vi "编码输出.vi"(8 "error in (no error)":errorcluster, 11 "SingleStepTestV3输入":refnum<class "SingleStepTestV2.lvclass">) -> (0 "error out":errorcluster, 3 "SingleStepTestV3输出":refnum<class "SingleStepTestV2.lvclass">)   [LabVIEW 2016, in "SingleStepTestV2.lvlib" / "SingleStepTestV2.lvclass"]
uses:
  SingleStepTestV2.lvclass
  SingleStepTestV2.lvclass/SingleStepTestV2.ctl
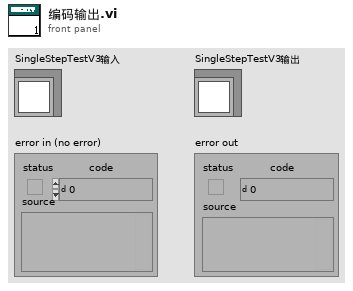
[diagram p1: front panel]
types:
  T1 = typedef "SingleStepTestV2.lvclass/State Data.ctl" = cluster{"data":u16[]}
  T2 = typedef "SingleStepTestV2.lvclass/控温操作.ctl" = enum32{"未选择", "控温开", "控温关"}
  T3 = typedef "SingleStepTestV3.lvclass/注射泵操作.ctl" = enum32{"复位", "注入", "注出", "等待"}
  T4 = typedef "SingleStepTestV2.lvclass/外设选择.ctl" = enum32{"未选择", "V1开", "V1关", "V2开", "V2关"}
  T5 = typedef "SingleStepTestV2.lvclass/外设选择2.ctl" = cluster{"V9-1":bool, "V9-2":bool}
  T6 = typedef "SingleStepTestV3.lvclass/项目输入.ctl" = u16
  T7 = typedef "SingleStepTestV2.lvclass/阀口操作.ctl" = enum32{"未选择", "V1", "V2", "V3", "V4", "V5", "V6", "V7", "V8", "V9", "V10", "V11", "V12"}
  T8 = typedef "SingleStepTestV2.lvclass/灯选择.ctl" = enum32{"未选择", "520", "660", "加热恒温", "氙灯/紫灯"}
  T9 = typedef "SingleStepTestV2.lvclass/ADC选择.ctl" = enum32{"未选择", "ADC0", "降温温度", "消解温度", "光谱/ADC1"}
  T10 = typedef "SingleStepTestV3.lvclass/数值输入.ctl" = i16
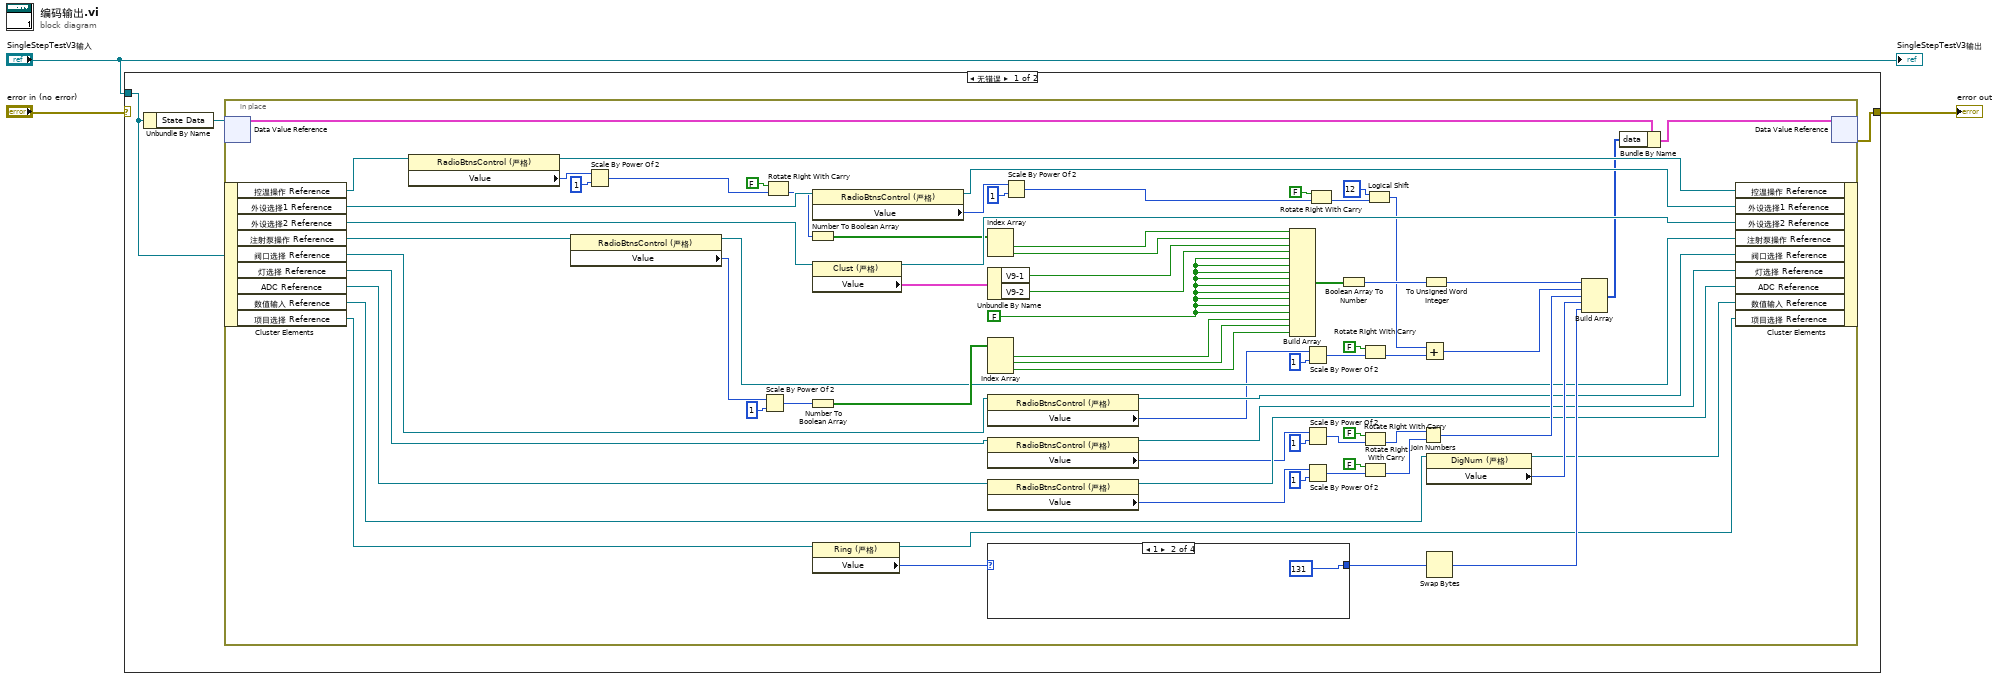
[diagram p0: block diagram]
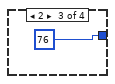
[diagram p3: hidden frame]
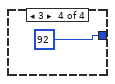
[diagram p4: hidden frame]
diagram:
  n1 = case shown="无错误" "error in (no error)" {
    selector: "error in (no error)" -> [_ w82]
    tunnel: "SingleStepTestV3输入" -> [w5 _]
    tunnel: [w4 w82] -> w3
    frame No Error {
      n2 = Unbundle By Name(w5) -> ("State Data"=w6:refnum<data-value>)
      n3 = in-place {
        w24 = FALSE
        n4 = in-place-dvr #1(w6) -> (w32:T1)  [unwired: 1 out]
        n5 = in-place-cluster #2(w5) -> ("控温操作 Reference"=w77:refnum<vi>, "外设选择1 Reference"=w72:refnum<vi>, "外设选择2 Reference"=w71:refnum<vi>, "注射泵操作 Reference"=w70:refnum<vi>, "阀口选择 Reference"=w66:refnum<vi>, "灯选择 Reference"=w64:refnum<vi>, "ADC Reference"=w63:refnum<vi>, "数值输入 Reference"=w60:refnum<vi>, "项目选择 Reference"=w59:refnum<vi>)
        n6 = property class="RadioBtnsControl (严格)"(reference=w77) -> (reference out=w50:refnum<vi>, "Value"=w23:T2)  [unwired: 1 in, 1 out]
        n7 = property class="RadioBtnsControl (严格)"(reference=w70) -> (reference out=w47:refnum<vi>, "Value"=w74:T3)  [unwired: 1 in, 1 out]
        n8 = Scale By Power Of 2(n=w23, x=u8 1) -> (x*2^n=w30:u8)
        n9 = Scale By Power Of 2(n=w74, x=u8 1) -> (x*2^n=w75:u8)
        n10 = Rotate Right With Carry(2:w30, 3:FALSE ("进位")) -> (0:w28:u8)  [unwired: 1 out]
        n11 = Number To Boolean Array(number=w28) -> (Boolean array=w27:bool[])
        n12 = Number To Boolean Array(number=w75) -> (Boolean array=w73:bool[])
        n13 = property class="RadioBtnsControl (严格)"(reference=w72) -> (reference out=w49:refnum<vi>, "Value"=w19:T4)  [unwired: 1 in, 1 out]
        n14 = property class="Clust (严格)"(reference=w71) -> (reference out=w48:refnum<vi>, "Value"=w11:T5)  [unwired: 1 in, 1 out]
        n15 = property class="Ring (严格)"(reference=w59) -> (reference out=w42:refnum<vi>, "Value"=w8:T6)  [unwired: 1 in, 1 out]
        n16 = Index Array(array=w27) -> (element #1=w26:bool, element #2=w25:bool)  [unwired: 2 in]
        n17 = Unbundle By Name(w11) -> ("V9-1"=w10:bool, "V9-2"=w9:bool)
        n18 = Index Array(array=w73) -> (element #1=w69:bool, element #2=w68:bool, element #3=w67:bool)  [unwired: 3 in]
        n19 = property class="RadioBtnsControl (严格)"(reference=w66) -> (reference out=w46:refnum<vi>, "Value"=w39:T7)  [unwired: 1 in, 1 out]
        n20 = property class="RadioBtnsControl (严格)"(reference=w64) -> (reference out=w45:refnum<vi>, "Value"=w33:T8)  [unwired: 1 in, 1 out]
        n21 = property class="RadioBtnsControl (严格)"(reference=w63) -> (reference out=w44:refnum<vi>, "Value"=w34:T9)  [unwired: 1 in, 1 out]
        n22 = case shown="1" w8 {
          selector: w8 -> [w78 _ _ _]
          tunnel: [w78 u16 131 ("Value") u16 76 ("Value") u16 92 ("Value")] -> w7
          frame 0, Default {
          }
          frame 1 {
          }
          frame 2 {
          }
          frame 3 {
          }
        }
        n23 = Scale By Power Of 2(n=w19, x=u16 1) -> (x*2^n=w21:u16)
        n24 = Build Array(w26, w25, w10, w9, w24, w24, w24, w24, w24, w24, w24, w24, w24, w69, w68, w67) -> (w56:bool[])
        n25 = Scale By Power Of 2(n=w39, x=u16 1) -> (x*2^n=w14:u16)
        n26 = Scale By Power Of 2(n=w33, x=u8 1) -> (x*2^n=w57:u8)
        n27 = Scale By Power Of 2(n=w34, x=u8 1) -> (x*2^n=w58:u8)
        n28 = Rotate Right With Carry(2:w21, 3:FALSE ("进位")) -> (0:w18:u16)  [unwired: 1 out]
        n29 = Boolean Array To Number(Boolean array=w56) -> (number=w55:u32)
        n30 = Rotate Right With Carry(2:w14, 3:FALSE ("进位")) -> (0:w13:u16)  [unwired: 1 out]
        n31 = Rotate Right With Carry(2:w57, 3:FALSE ("进位")) -> (0:w38:u8)  [unwired: 1 out]
        n32 = Rotate Right With Carry(2:w58, 3:FALSE ("进位")) -> (0:w36:u8)  [unwired: 1 out]
        n33 = Logical Shift(y=i16 12, x=w18) -> (x << y=w16:u16)
        n34 = Join Numbers(hi=w38, lo=w36) -> ((hi.lo)=w54:u16)
        n35 = Add(x=w16, y=w13) -> (x+y=w12:u16)
        n36 = To Unsigned Word Integer(number=w55) -> (unsigned 16bit integer=w51:u16)
        n37 = property class="DigNum (严格)"(reference=w60) -> (reference out=w43:refnum<vi>, "Value"=w53:T10)  [unwired: 1 in, 1 out]
        n38 = Swap Bytes(anything=w7) -> (byte swapped=w52:T6)
        n39 = Build Array(w51, w12, w54, w53, w52) -> (w40:T6[])
        n40 = Bundle By Name(cluster=w32, "data"=w40) -> (w41:T1)
        n41 = in-place-cluster #2("控温操作 Reference"=w50, "外设选择1 Reference"=w49, "外设选择2 Reference"=w48, "注射泵操作 Reference"=w47, "阀口选择 Reference"=w46, "灯选择 Reference"=w45, "ADC Reference"=w44, "数值输入 Reference"=w43, "项目选择 Reference"=w42) -> ()  [unwired: 1 out]
        n42 = in-place-dvr #1(w41) -> (w4:errorcluster)  [unwired: 1 out]
      }
    }
    frame Error {
    }
  }
  "error out" <- w3
  "SingleStepTestV3输出" <- "SingleStepTestV3输入"
